vi "Vision Logic New.vi"(8 "Y Default/Base Value":sgl, 9 "Y Coordinate of the Box":sgl=-1.0, 10 "X Default/Base Value":sgl, 11 "X Coordinate of the Box":sgl=-1.0) -> ()   [LabVIEW 2016]
uses:
  <vilib>/Rock Robotics/WPI/Utilities/WPI_GetSetVariantRefNum.vi
  <vilib>/Rock Robotics/WPI/RobotDrive/WPI_RobotDriveArcadeDrive_Standard(NoSaturation).vi
  <vilib>/Rock Robotics/WPI/Ultrasonic/WPI_SonarMB1010AnalogRefNum Registry Get.vi
  <vilib>/Rock Robotics/WPI/Ultrasonic/WPI_SonarMB1010AnalogGetRange.vi
  LabVIEW Data/Zeus Dashboard/VisionProcessingBoolean.vi
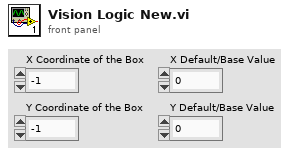
[diagram p1: front panel]
types:
  T1 = typedef "WPI_RobotDriveDevRef.ctl" = cluster{"DevStatus":errorcluster, "Motors[]":T2[], "Square Inputs":bool, "Max Output":dbl}
  T2 = typedef "WPI_MotorControlDeviceRef.ctl" = cluster{"DeviceStatus":errorcluster, "Type":T3, "PWM":cluster{"PWM Channel":T4, "DeadBand":T5}, "CAN":cluster{"Device Number":u8, "SetOutput VI Ref":variant, "GetOutput VI Ref":variant, "Enable VI Ref":variant, "Disable VI Ref":variant, "Data":variant}, "Invert":bool}
  T3 = typedef "WPI_MotorControlType.ctl" = enum16{"PWM", "CAN"}
  T4 = typedef "FPGA_DIOPWMChannel.ctl" = enum8{"PWM 0", "PWM 1", "PWM 2", "PWM 3", "PWM 4", "PWM 5", "PWM 6", "PWM 7", "PWM 8", "PWM 9", "PWM MXP 0", "PWM MXP 1", "PWM MXP 2", "PWM MXP 3", "PWM MXP 4", "PWM MXP 5", "PWM MXP 6", "PWM MXP 7", "PWM MXP 8", "PWM MXP 9", "Invalid"}
  T5 = typedef "WPI_PWMDeadband.ctl" = cluster{"Name":string, "maxPositivePwm":i32, "minPositivePwm":i32, "centerPwm":i32, "maxNegativePwm":i32, "minNegativePwm":i32, "angularRange":u16}
  T6 = typedef "WPI_SonarMB1010AnalogDeviceRef.ctl" = cluster{"AIDeviceRef":T7, "Scaling factor (V/in)":dbl, "Average Bits":u8}
  T7 = typedef "WPI_AnalogChannelDevRef.ctl" = cluster{"DevStatus":errorcluster, "Analog Channel":T8}
  T8 = typedef "FPGA_AIChannel.ctl" = enum8{"AI 0", "AI 1", "AI 2", "AI 3", "AI MXP 0", "AI MXP 1", "AI MXP 2", "AI MXP 3", "Invalid"}
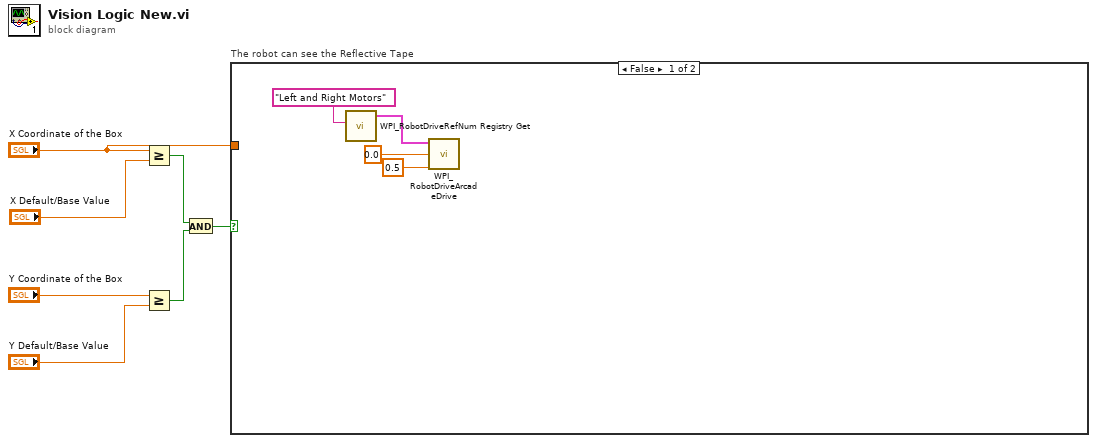
[diagram p0: block diagram]
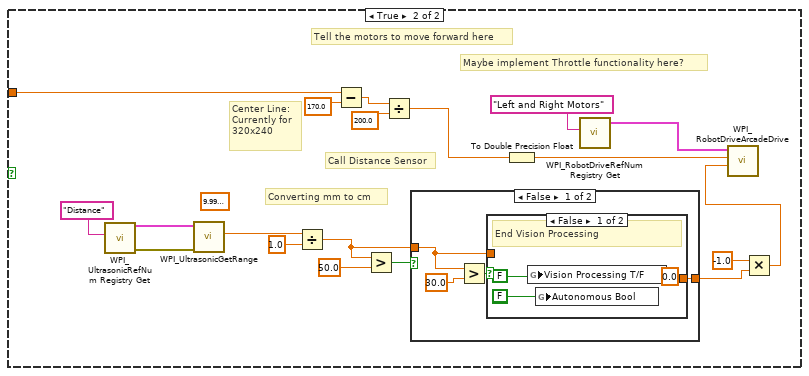
[diagram p2: hidden frame]
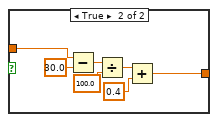
[diagram p3: hidden frame]
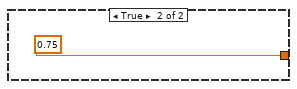
[diagram p4: hidden frame]
diagram:
  n1 = Greater Or Equal?(x="X Coordinate of the Box", y="X Default/Base Value") -> (x >= y?=w4:bool)
  n2 = Greater Or Equal?(x="Y Coordinate of the Box", y="Y Default/Base Value") -> (x >= y?=w3:bool)
  n3 = And(x=w4, y=w3) -> (x .and. y?=w2:bool)
  n4 = case "The robot can see the Reflective Tape" shown="False" w2 {
    tunnel: "X Coordinate of the Box" -> [_ w21]
    frame False {
      n5 = call <vilib>:"WPI_RobotDriveRefNum Registry Get.vi"("refnum name"="Left and Right Motors") -> ("RobotDriveDevRef"=w8:T1)  [unwired: 9 in, 1 out]
      n6 = call-poly <vilib>:"WPI_RobotDriveArcadeDrive.vi"("Y axis value"=0.5, "X axis value"=0.0, "RobotDriveDevRef"=w8) -> ()  [unwired: 6 in, 3 out]
    }
    frame True {
      (unwired) sgl 1e-05 ("ping time (s)")
      # "Center Line: Currently for 320x240"
      # "Converting mm to cm"
      # "Call Distance Sensor"
      # "Maybe implement Throttle functionality here?"
      # "Tell the motors to move forward here"
      n7 = call-poly <vilib>:"WPI_UltrasonicRefNum Registry Get.vi"("refnum name"="Distance") -> ("error out"=w17:errorcluster, "SonarMB1010AnalogDevRef"=w18:T6)  [unwired: 9 in]
      n8 = call-poly <vilib>:"WPI_UltrasonicGetRange.vi"("error in"=w17, "SonarMB1010AnalogDevRef"=w18) -> ("Distance"=w16:dbl)  [unwired: 7 in, 2 out]
      n9 = Divide(x=w16, y=1.0) -> (x/y=w22:dbl)
      n10 = Subtract(x=w21, y=sgl 170.0) -> (x-y=w29:sgl)
      n11 = Greater?(x=w22, y=50.0) -> (0:w24:bool)
      n12 = Divide(x=w29, y=sgl 200.0) -> (x/y=w20:sgl)
      n13 = case shown="False" w24 {
        tunnel: [w34 0.75] -> w13
        tunnel: w22 -> [w33 _]
        frame False {
          n14 = Greater?(x=w33, y=30.0) -> (0:w31:bool)
          n15 = case shown="False" w31 {
            tunnel: w33 -> [_ w44]
            tunnel: [0.0 w38] -> w34
            frame False {
              (unwired) FALSE ("Vision Processing T/F")
              # "End Vision Processing"
              n16 = global write "VisionProcessingBoolean.vi" "Vision Processing T/F"(FALSE ("Vision Processing T/F")) -> ()
              n17 = global write "VisionProcessingBoolean.vi" "Autonomous Bool"(TRUE ("Vision Processing T/F")) -> ()
            }
            frame True {
              n18 = Subtract(x=w44, y=30.0) -> (x-y=w42:dbl)
              n19 = Divide(x=w42, y=100.0) -> (x/y=w40:dbl)
              n20 = Add(x=w40, y=0.4) -> (x+y=w38:dbl)
            }
          }
        }
        frame True {
        }
      }
      n21 = To Double Precision Float(number=w20) -> (double precision float=w19:dbl)
      n22 = call <vilib>:"WPI_RobotDriveRefNum Registry Get.vi"("refnum name"="Left and Right Motors") -> ("RobotDriveDevRef"=w26:T1)  [unwired: 9 in, 1 out]
      n23 = Multiply(x=-1.0, y=w13) -> (x*y=w14:dbl)
      n24 = call-poly <vilib>:"WPI_RobotDriveArcadeDrive.vi"("Y axis value"=w14, "X axis value"=w19, "RobotDriveDevRef"=w26) -> ()  [unwired: 6 in, 3 out]
    }
  }
